vi "Step Update Table 5.0 to 5.1.vi"(8 "error in (no error)":errorcluster, 11 "Connection Refnum":T1) -> (0 "error out":errorcluster, 3 "Connection Refnum":T1)   [LabVIEW 2011]
uses:
  Summitek EXT/ODBC/SQL Controls/Connection Refnum.ctl
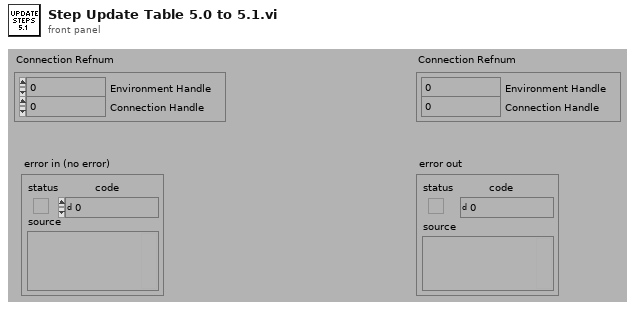
[diagram p1: front panel]
types:
  T1 = typedef "Connection Refnum.ctl" = cluster{"Environment Handle":i32, "Connection Handle":i32}
  T2 = typedef "Step Record.ctl" = cluster{"ixStep":i32, "sxSequenceId":string, "sxTestId":string, "iIndex":i32, "iRepeat":i32, "iQuickMode":i32, "sTag":string, "sDatasheetsCSV":string, "bConfiguration":string}
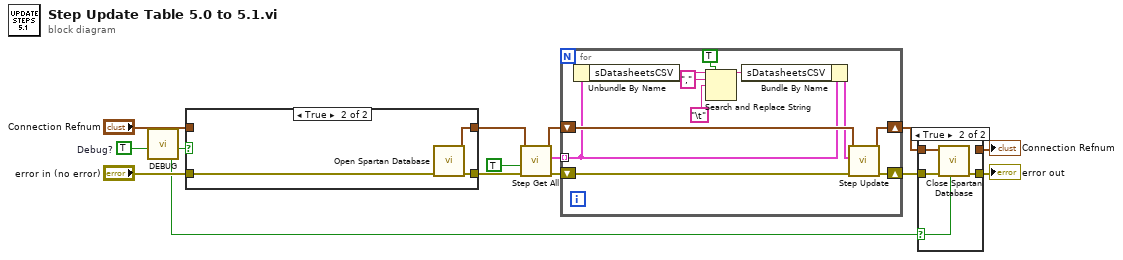
[diagram p0: block diagram]
diagram:
  w11 = TRUE  # Debug?
  n1 = call "DEBUG.vi"("Dev DEBUG? (f)"=w11) -> ("DEBUG?"=w9:bool)  [unwired: 1 in, 5 out]
  n2 = case shown="True" w9 {
    tunnel: "Connection Refnum" -> [w16 _]
    tunnel: "error in (no error)" -> [w15 w19]
    tunnel: [w15 w18] -> w4
    tunnel: [w16 w17] -> w8
    frame False {
    }
    frame True {
      n3 = call "Open Spartan Database.vi"("error in (no error)"=w19) -> ("error out"=w18:errorcluster, "Connection Refnum"=w17:T1)  [unwired: 2 in, 7 out]
    }
  }
  n4 = call "Step Get All.vi"("error in (no error)"=w4, "All Steps? (f)"=TRUE, "Connection Refnum"=w8) -> ("error out"=w7:errorcluster, "Sequence Steps"=w5:T2[], "Connection Refnum"=w6:T1)  [unwired: 2 in, 4 out]
  n5 = for {
    shift-right: [w27] -> w2
    shift-left: w7 -> [w28]
    shift-right: [w26] -> w1
    shift-left: w6 -> [w29]
    tunnel: w5 -> [w25] mode=indexing
    n6 = Unbundle By Name(w25) -> ("sDatasheetsCSV"=w30:string)
    n7 = Search and Replace String(replace all?=TRUE ("replace all? (F)"), input string=w30, search string=",", replace string="\t") -> (result string=w22:string)  [unwired: 1 in, 6 out]
    n8 = Bundle By Name(cluster=w25, "sDatasheetsCSV"=w22) -> (w24:T2)
    n9 = call "Step Update.vi"("error in (no error)"=w28, "Step Record (empty)"=w24, "Connection Refnum"=w29) -> ("error out"=w27:errorcluster, "Connection Refnum"=w26:T1)  [unwired: 7 out]
  }
  n10 = case shown="True" w9 {
    selector: w9 -> [_ w33]
    tunnel: w2 -> [w32 w36]
    tunnel: [w31 _] -> w10
    tunnel: [w32 w35] -> w12
    tunnel: w1 -> [w31 w34]
    frame False {
    }
    frame True {
      n11 = call "Close Spartan Database.vi"("Force Close? (f)"=w33, "error in (no error)"=w36, "Connection Refnum"=w34) -> ("error out"=w35:errorcluster)  [unwired: 2 in, 6 out]
    }
  }
  "Connection Refnum" <- w10
  "error out" <- w12
